vi "DrawVessels.vi"(8 "error in (no error)":errorcluster, 11 "Image in":refnum<class "Image.lvclass">) -> (0 "error out":errorcluster, 3 "Image out":refnum<class "Image.lvclass">)   [LabVIEW 2013, in "Image.lvclass"]
uses:
  Image.lvclass
  Image.lvclass/Image.ctl
  <vilib>/vision/NI_Vision_Development_Module.lvlib
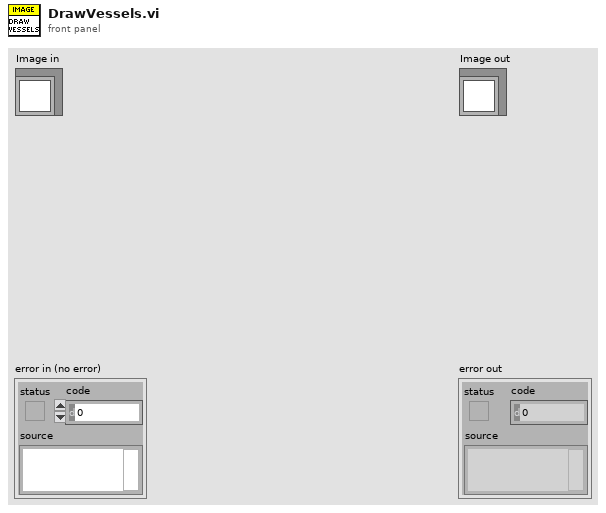
[diagram p1: front panel]
types:
  T1 = typedef "IMAQ Image.ctl" = refnum<image>
  T2 = cluster{"scan_idx":i32, "lens":i32, "mag":dbl, "x":dbl, "y":dbl, "mouse_id":i32, "exp_date":string, "file_name":string, "file_path":path}
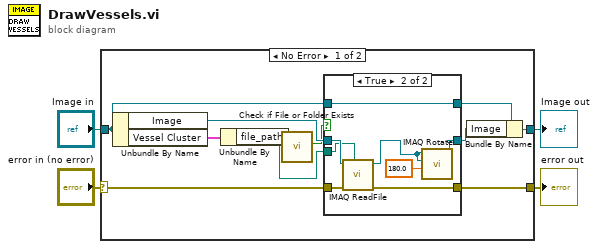
[diagram p0: block diagram]
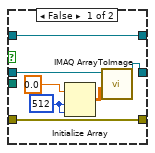
[diagram p2: hidden frame]
diagram:
  n1 = case shown="No Error" "error in (no error)" {
    selector: "error in (no error)" -> [w13 w31]
    tunnel: [w12 w31] -> w3
    tunnel: [w6 w30] -> w1
    tunnel: "Image in" -> [w9 w30]
    frame No Error {
      n2 = Unbundle By Name(w9) -> ("Image"=w14:T1, "Vessel Cluster"=w8:T2)
      n3 = Unbundle By Name(w8) -> ("file_path"=w10:path)
      n4 = call <vilib>:"Check if File or Folder Exists.vi"("path"=w10) -> ("file or folder exists?"=w11:bool)  [unwired: 8 in, 2 out]
      n5 = case shown="True" w11 {
        tunnel: w14 -> [w17 w29]
        tunnel: w13 -> [w20 w28]
        tunnel: [w20 w27] -> w12
        tunnel: w10 -> [_ w26]
        tunnel: w9 -> [w21 w25]
        tunnel: [w21 w25] -> w7
        tunnel: [w15 w22] -> w5
        frame False {
          w18 = 512 ("dimension size")
          n6 = Initialize Array(0.0 ("element"), w18, w18) -> (w16:dbl[][])
          n7 = call "IMAQ ArrayToImage"("Image Pixels (I16)"=w16, "Image"=w17) -> ("Image Out"=w15:T1)  [unwired: 8 in, 1 out]
        }
        frame True {
          n8 = call "IMAQ ReadFile"("File Path"=w26, "error in (no error)"=w28, "Image"=w29) -> ("error out"=w27:errorcluster, "Image Out"=w23:T1)  [unwired: 2 in, 5 out]
          n9 = call "IMAQ Rotate"("Angle (degrees)"=sgl 180.0, "Image Dst"=w23, "Image Src"=w23) -> ("Image Dst Out"=w22:T1)  [unwired: 7 in, 1 out]
        }
      }
      n10 = Bundle By Name(cluster=w7, "Image"=w5) -> (w6:refnum<class "Image.lvclass">)
    }
    frame Error {
    }
  }
  "error out" <- w3
  "Image out" <- w1
